vi "IlluminatedG_ApplyLibraryIconToVIs.vi"(11 "Library":refnum<vi>) -> (0 "error out":errorcluster)   [LabVIEW 2022 SP3]
uses:
  <vilib>/LabVIEW Icon API/lv_icon/Controls/LayerType.ctl
  <vilib>/LabVIEW Icon API/lv_icon/Controls/Layer.ctl
  <vilib>/LabVIEW Icon API/lv_icon/Classes/Layer/Layer.lvclass
  <vilib>/LabVIEW Icon API/lv_icon/Classes/Icon/Icon.lvclass
  <vilib>/LabVIEW Icon API/LabVIEW Icon API.lvlib
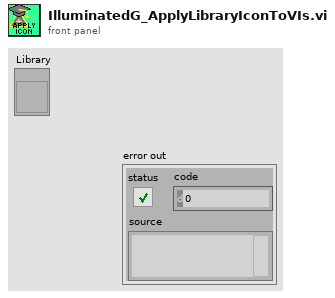
[diagram p1: front panel]
types:
  T1 = typedef "imagedata.ctl" = cluster{"image type":i32, "image depth":i32, "image":u8[], "mask":u8[], "colors":u32[], "Rectangle":cluster{"left":i16, "top":i16, "right":i16, "bottom":i16}}
  T2 = typedef "Layer.ctl" = cluster{"LayerIcon":picture, "LayerName":string, "Opacity":u8, "Visibility?":bool}
  T3 = typedef "LayerType.ctl" = enum16{"Graphic", "Text", "Tool", "Graphic Drop"}
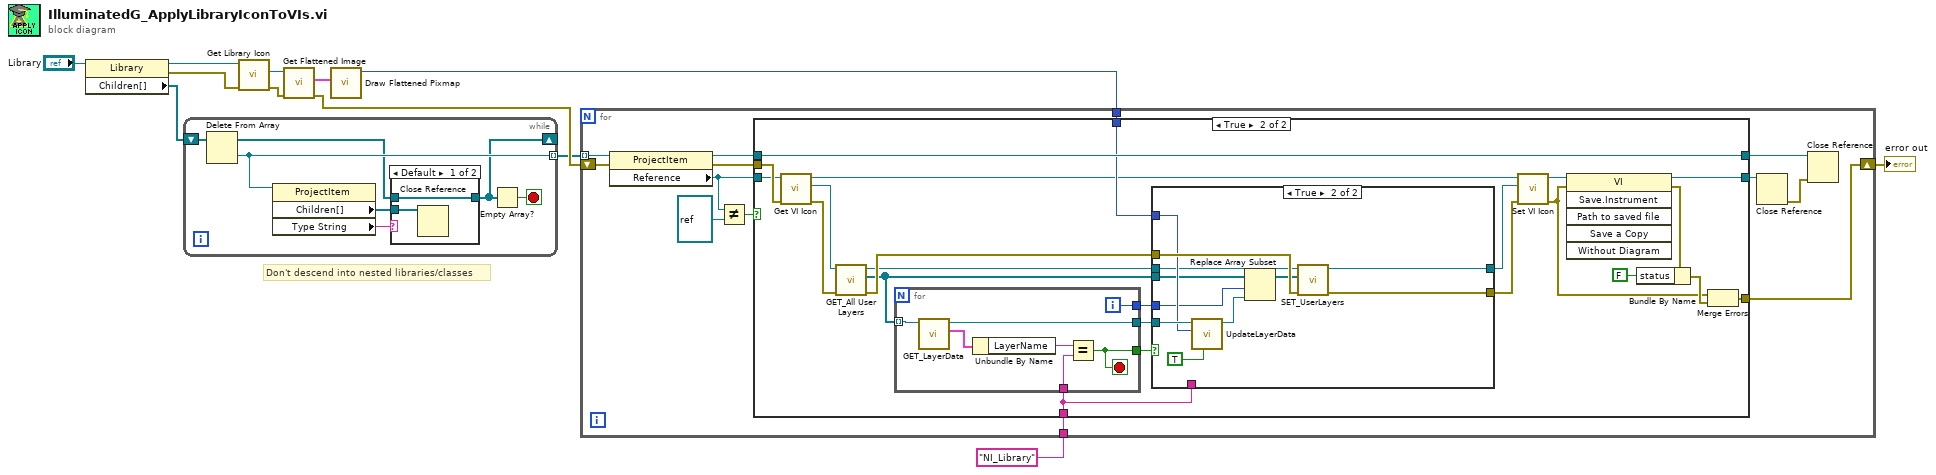
[diagram p0: block diagram]
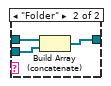
[diagram p2: hidden frame]
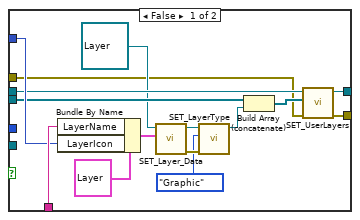
[diagram p4: hidden frame]
diagram:
  # "Don't descend into nested libraries/classes"
  n1 = property class="Library"(reference="Library") -> (reference out=w9:refnum<vi>, error out=w3:errorcluster, "Children[]"=w10:refnum<vi>[])  [unwired: 1 in]
  n2 = while {
    shift-right: [w14] -> _
    shift-left: w10 -> [w19]
    tunnel: [w17] -> w7 mode=indexing
    stop <- w18 stop-if-true
    n3 = Delete From Array(array=w19) -> (deleted portion=w17:refnum<vi>, array with subset deleted=w16:refnum<vi>[])  [unwired: 2 in]
    n4 = property class="ProjectItem"(reference=w17) -> ("Children[]"=w15:refnum<vi>[], "Type String"=w13:string)  [unwired: 1 in, 2 out]
    n5 = case shown="Default" w13 {
      tunnel: w16 -> [w21 w24]
      tunnel: w15 -> [w20 w23]
      tunnel: [w21 w22] -> w14
      frame Default {
        n6 = Close Reference(reference=w20) -> ()  [unwired: 1 in, 1 out]
      }
      frame "Folder" {
        n7 = Build Array (concatenate)(w24, w23) -> (w22:refnum<vi>[])
      }
    }
    n8 = Empty Array?(array=w14) -> (empty?=w18:bool)
  }
  n9 = call <vilib>:"Get Library Icon.vi"("error in (no error)"=w3, "Library Refnum in"=w9) -> ("error out"=w2:errorcluster, "Icon"=w11:refnum<class "Icon.lvclass">)  [unwired: 7 in, 1 out]
  n10 = call <vilib>:"Get Flattened Image.vi"("error in (no error)"=w2, "lv_icon.lvlib:Icon.lvclass in"=w11) -> ("error out"=w12:errorcluster, "Color Image"=w6:T1)  [unwired: 6 in, 2 out]
  n11 = call <vilib>:"Draw Flattened Pixmap.vi"("image data"=w6) -> ("new picture"=w5:picture)  [unwired: 8 in]
  n12 = for {
    tunnel: "NI_Library" -> [w30]
    tunnel: w7 -> [w29] mode=indexing
    tunnel: w5 -> [w28]
    shift-right: [w25] -> w1
    shift-left: w12 -> [w27]
    n13 = property class="ProjectItem"(reference=w29, error in=w27) -> (reference out=w35:refnum<vi>, error out=w26:errorcluster, "Reference"=w32:refnum<vi>)
    n14 = Not Equal?(x=w32, y=refnum<vi> refnum) -> (x != y?=w36:bool)
    n15 = case shown="True" w36 {
      tunnel: w35 -> [w40 w59]
      tunnel: [w40 w59] -> w34
      tunnel: [w39 w48] -> w33
      tunnel: w32 -> [w39 w61]
      tunnel: w30 -> [_ w52]
      tunnel: w28 -> [_ w53]
      tunnel: w26 -> [w38 w62]
      tunnel: [w38 w41] -> w25
      frame False {
      }
      frame True {
        n16 = call <vilib>:"Get VI Icon.vi"("error in (no error)"=w62, "VI Refnum in"=w61) -> ("error out"=w47:errorcluster, "Icon"=w60:refnum<class "Icon.lvclass">, "VI Refnum out"=w51:refnum<vi>)  [unwired: 7 in]
        n17 = call-dynamic "GET_All User Layers.vi"("error in (no error)"=w47, "Icon.lvclass in"=w60) -> ("error out"=w63:errorcluster, "User Layer"=w54:refnum<class "Layer.lvclass">[], "Icon.lvclass out"=w58:refnum<class "Icon.lvclass">)  [unwired: 7 in]
        n18 = for {
          tunnel: w54 -> [w70] mode=indexing
          tunnel: w52 -> [w68]
          tunnel: [w67] -> w57
          tunnel: [w66] -> w55
          tunnel: [w65] -> w56
          i -> [w65]
          stop <- w66 stop-if-true
          n19 = call-dynamic "GET_LayerData.vi"("Layer.lvclass in"=w70) -> ("Data"=w69:T2, "Layer.lvclass out"=w67:refnum<class "Layer.lvclass">)  [unwired: 6 in, 3 out]
          n20 = Unbundle By Name(w69) -> ("LayerName"=w64:string)
          n21 = Equal?(x=w64, y=w68) -> (x = y?=w66:bool)
        }
        n22 = case shown="True" w55 {
          tunnel: w58 -> [w75 w90]
          tunnel: w57 -> [_ w95]
          tunnel: w56 -> [_ w91]
          tunnel: w54 -> [w77 w93]
          tunnel: w53 -> [w78 w94]
          tunnel: [w74 w88] -> w49
          tunnel: w52 -> [w81 _]
          tunnel: w63 -> [w72 w96]
          tunnel: [w71 w87] -> w46
          frame False {
            n23 = Bundle By Name(cluster=T2 {"LayerIcon"=bytes[3102], "LayerName"="", "Opacity"=100, "Visibility?"=TRUE} ("Data"), "LayerName"=w81, "LayerIcon"=w78) -> (w79:T2)
            n24 = call-dynamic "SET_Layer_Data.vi"("Data"=w79, "Layer.lvclass in"=refnum<class "Layer.lvclass"> refnum) -> ("error out"=w84:errorcluster, "Layer.lvclass out"=w83:refnum<class "Layer.lvclass">)  [unwired: 2 in, 6 out]
            n25 = call-dynamic "SET_LayerType.vi"("error in (no error)"=w84, "Type"=LayerType."Graphic", "Layer.lvclass in"=w83) -> ("Layer.lvclass out"=w76:refnum<class "Layer.lvclass">)  [unwired: 8 out]
            n26 = Build Array (concatenate)(w77, w76) -> (w85:refnum<class "Layer.lvclass">[])
            n27 = call-dynamic "SET_UserLayers.vi"("error in (no error)"=w72, "Layers"=w85, "Icon.lvclass in"=w75) -> ("error out"=w71:errorcluster, "Icon.lvclass out"=w74:refnum<class "Icon.lvclass">)  [unwired: 7 in]
          }
          frame True {
            n28 = call <vilib>:"UpdateLayerData.vi"("Overwrite?"=TRUE, "new picture"=w94, "Active Layer"=w95) -> ("Layer.lvclass out"=w92:refnum<class "Layer.lvclass">)  [unwired: 7 in, 1 out]
            n29 = Replace Array Subset(array=w93, new element=w92, index=w91) -> (w89:refnum<class "Layer.lvclass">[])
            n30 = call-dynamic "SET_UserLayers.vi"("error in (no error)"=w96, "Layers"=w89, "Icon.lvclass in"=w90) -> ("error out"=w87:errorcluster, "Icon.lvclass out"=w88:refnum<class "Icon.lvclass">)  [unwired: 7 in]
          }
        }
        n31 = call <vilib>:"Set VI Icon.vi"("error in (no error)"=w46, "Icon"=w49, "VI Refnum in"=w51) -> ("error out"=w42:errorcluster, "VI Refnum out"=w50:refnum<vi>)  [unwired: 7 in]
        n32 = invoke class="VI" method="Save.Instrument"(reference=w50, error in=w42) -> (reference out=w48:refnum<vi>, error out=w45:errorcluster)  [unwired: 4 in, 4 out]
        n33 = Bundle By Name(cluster=w45, "status"=FALSE) -> (w43:errorcluster)
        n34 = Merge Errors(w42, w43) -> (w41:errorcluster)
      }
    }
    n35 = Close Reference(reference=w33) -> (error out=w31:errorcluster)  [unwired: 1 in]
    n36 = Close Reference(reference=w34, error in (no error)=w31) -> ()  [unwired: 1 out]
  }
  "error out" <- w1
